vi "TX_双音扫频IMD3.vi"() -> ()   [LabVIEW 2015]
uses:
  <vilib>/Instr/_visa.llb/VISA Configure Serial Port (Instr).vi
  <instrlib>/Agilent E363X Series/Agilent E363X Series.lvlib
  <instrlib>/Rohde&Schwarz Spectrum Analyzer/Rohde&Schwarz Spectrum Analyzer.lvlib
panel:
  out "VISA resource name out 2":refnum<visa-resource-name>
  out "VISA resource name out":refnum<visa-resource-name>
  in  "Stop Frequency (0.0) 2":dbl=2130000000.0 caption="Stop Frequency (0.0)" format="%#.9p"
  in  "Start Frequency (0.0) 2":dbl=2000000000.0 caption="Start Frequency (0.0)" format="%#.9p"
  in  "Stop Frequency (0.0)":dbl=2130000000.0 format="%#.9p"
  in  "Start Frequency (0.0)":dbl=2000000000.0 format="%#.9p"
  in  "模板路径 2":path=path "E:/Everst_TestReport/Everst_TestReport_Template.xlsx"
  in  "测试板编号 2":i32=4
  in  "保存路径 2":path=path "E:/Everst_TestReport/Report/Everrst_#"
  in  "开关":bool[](array[boolean])=[FALSE, TRUE, FALSE, TRUE, FALSE, FALSE, FALSE, TRUE, TRUE, FALSE]
  in  "volt2v":dbl[](array[numeric])
  in  "volt1v3":dbl[](array[numeric])
  in  "error in (no error) 6":errorcluster {"code" format="%.0x"}
  in  "error in (no error) 5":errorcluster caption="error in (no error)"
  in  "error in (no error) 4":errorcluster caption="error in (no error)"
  in  "error in (no error) 3":errorcluster
  in  "error in (no error) 2":errorcluster
  in  "error in (no error)":errorcluster
  in  "直流电源2v":refnum<visa-resource-name>="GPIB0::6::INSTR"
  in  "Frequency (1.0e9 Hz)":dbl=10000000.0 format="%.3f"
  in  "RF Output Level (-30.0 dBm)":dbl=10.0 caption="RF Output Level (-30.0)" format="%.3f"
  in  "Reference Level Offset (0.0) 2":dbl=0.95 caption="Reference Level Offset (0.0)" format="%^.3e"
  in  "Coupling Value (0.0) 2":dbl=2000.0 caption="Coupling Value (0.0)" format="%^.3e"
  in  "Reference Level (-20.0) 2":dbl=30.0 caption="Reference Level (-20.0)" format="%^.3e"
  in  "Span (0.0) 2":dbl=1000000000.0 caption="Span (0.0)" format="%.1f"
  in  "Center Frequency (0.0) 2":dbl=2100000000.0 caption="Center Frequency (0.0)" format="%#.9p"
  in  "Reference Level Offset (0.0)":dbl=2.3 format="%^.3e"
  in  "Coupling Value (0.0)":dbl=2000.0 format="%^.3e"
  in  "Reference Level (-20.0)":dbl=30.0 format="%^.3e"
  in  "Span (0.0)":dbl=1000000000.0 format="%.1f"
  in  "Center Frequency (0.0)":dbl=2100000000.0 format="%#.9p"
  in  "配置文件路径":path=path "E:/Everst_TestReport/config.xlsx"
  out "Bamp_next":dbl[](array[numeric])
  out "Bamp_max":dbl[](array[numeric])
  in  "Marker Search 4":i32(ring)=1 caption="Marker Search" items=["Peak Maximum"=1, "Peak Minimum"=2, "Next Maximum"=3, "Left Maximum"=4, "Right Maximum"=5, "Next Minimum"=6, "Left Minimum"=7, "Right Minimum"=8]
  in  "Peak Excursion 4":dbl=3.0 caption="Peak Excursion" format="%.1f"
  out "channelB_y1":dbl[](array[numeric]) caption="Amplitude" format="%^.3e"
  out "channelB_x1":dbl[](array[numeric]) caption="X" format="%^.3e"
  out "Apos_next":dbl[](array[numeric])
  in  "Aamp_next":dbl[](array[numeric])
  out "Aamp_max":dbl[](array[numeric])
  out "Apos_max":dbl[](array[numeric])
  in  "Marker Search 3":i32(ring)=1 caption="Marker Search" items=["Peak Maximum"=1, "Peak Minimum"=2, "Next Maximum"=3, "Left Maximum"=4, "Right Maximum"=5, "Next Minimum"=6, "Left Minimum"=7, "Right Minimum"=8]
  in  "Peak Excursion 3":dbl=3.0 caption="Peak Excursion" format="%.1f"
  out "channelA_y1":dbl[](array[numeric]) caption="Amplitude" format="%^.3e"
  out "channelA_x1":dbl[](array[numeric]) caption="X" format="%^.3e"
  in  "信号发生器地址":refnum<visa-resource-name>="GPIB0::10::INSTR"
  in  "频谱仪地址B":refnum<visa-resource-name>="TCPIP0::192.168.1.4::inst0::INSTR"
  in  "频谱仪地址A":refnum<visa-resource-name>="GPIB0::22::INSTR"
  in  "直流电源(1.3V)":refnum<visa-resource-name>="GPIB0::4::INSTR"
  in  "FPGA串口地址":refnum<visa-resource-name>="COM3"
  out "fin":dbl[](array[numeric])
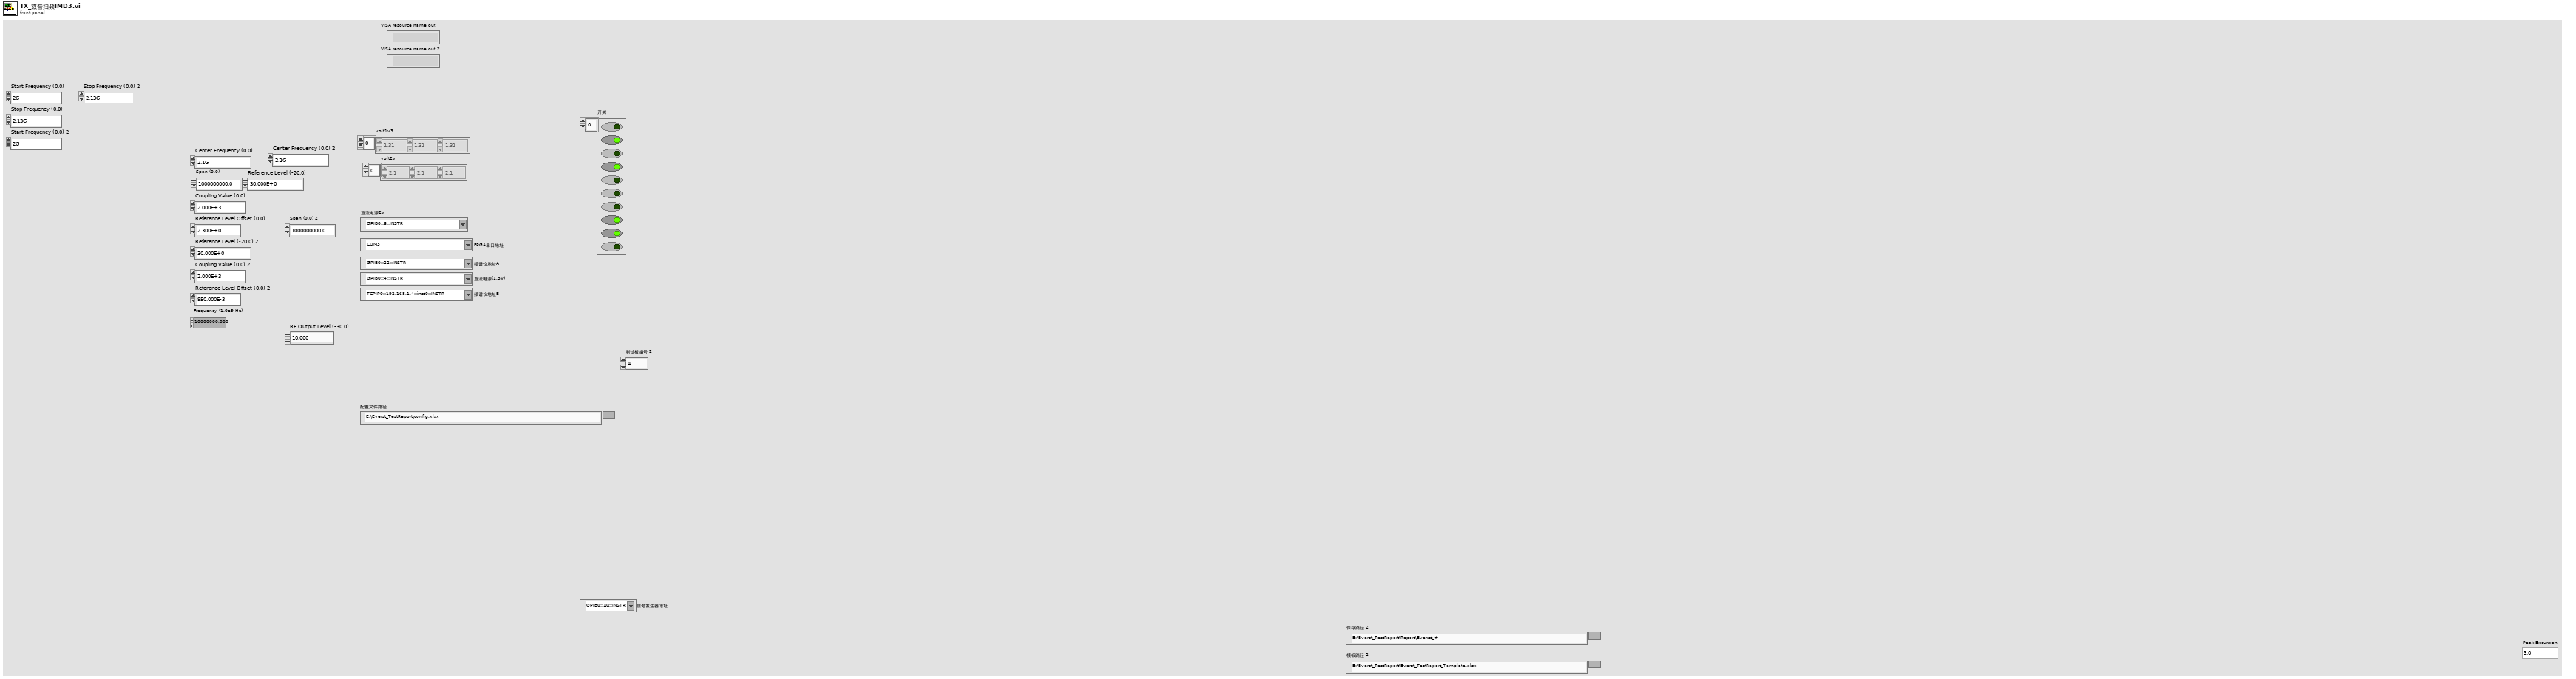
[diagram p1: front panel]
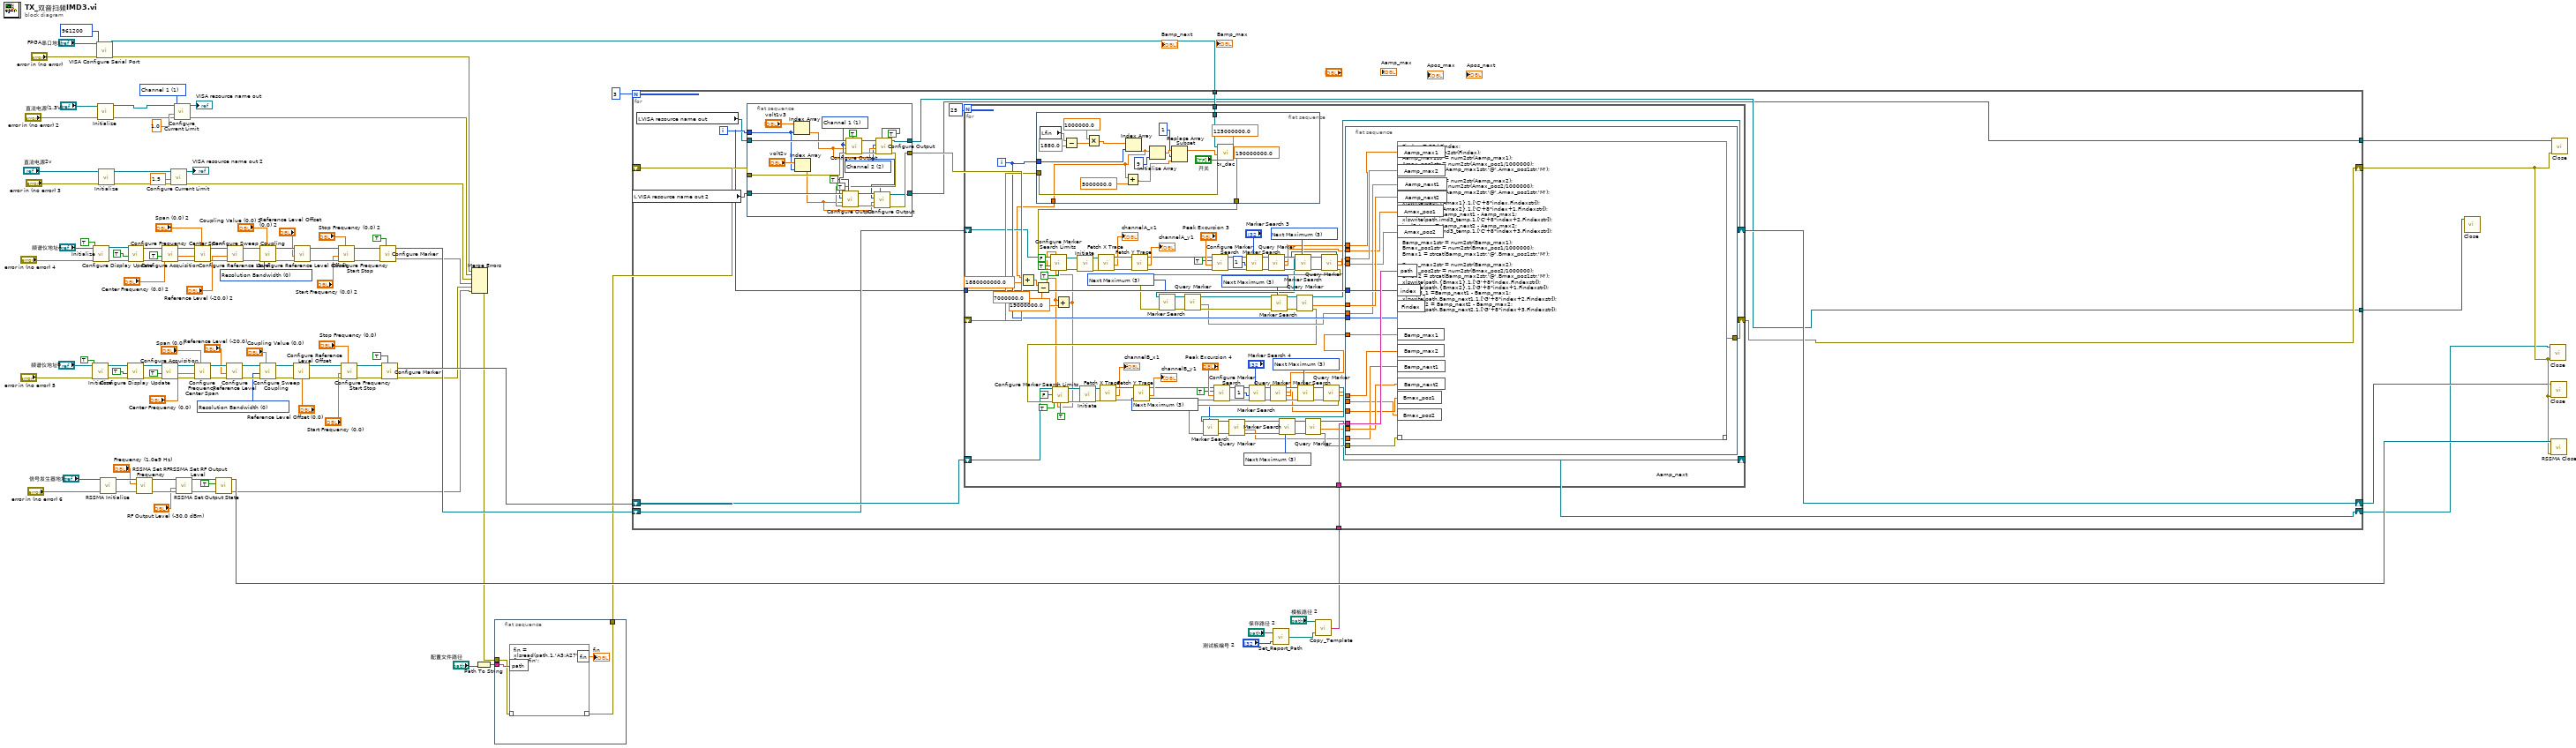
[diagram p0: block diagram]
diagram:
  w42 = 1 items=["Channel 1"=1, "Channel 2"=2, "Channel 3"=3] ("Channel (1: Channel 1)")
  w50 = 0 items=["Resolution Bandwidth", "Video Bandwidth", "Sweep Time"] ("Sweep Coupling (Resolution Bandwidth)")
  w72 = 0 items=["Resolution Bandwidth", "Video Bandwidth", "Sweep Time"] ("Sweep Coupling (Resolution Bandwidth)")
  n1 = call <instrlib>:"Initialize.vi"("VISA resource name"="频谱仪地址B", "Reset (T: Reset)"=TRUE, "error in (no error)"="error in (no error) 5") -> ("VISA resource name out"=w88:refnum<visa-resource-name>, "error out"=w89:errorcluster)  [unwired: 11 in]
  n2 = call <instrlib>:"Initialize.vi"("VISA resource name"="频谱仪地址A", "Reset (T: Reset)"=TRUE, "error in (no error)"="error in (no error) 4") -> ("VISA resource name out"=w66:refnum<visa-resource-name>, "error out"=w67:errorcluster)  [unwired: 11 in]
  n3 = call-poly "VISA Configure Serial Port"("VISA resource name"="FPGA串口地址", "baud rate (9600)"=u32 961200, "error in (no error)"="error in (no error)") -> ("VISA resource name out"=w111:refnum<visa-resource-name>, "error out"=w36:errorcluster)  [unwired: 11 in]
  n4 = call <instrlib>:"Initialize.vi"("error in (no error)"="error in (no error) 2", "VISA resource name"="直流电源(1.3V)") -> ("error out"=w39:errorcluster, "VISA resource name out"=w40:refnum<visa-resource-name>)  [unwired: 8 in]
  n5 = call <instrlib>:"Initialize.vi"("error in (no error)"="error in (no error) 3", "VISA resource name"="直流电源2v") -> ("error out"=w47:errorcluster, "VISA resource name out"=w46:refnum<visa-resource-name>)  [unwired: 8 in]
  n6 = call <instrlib>:"RSSMA Initialize.vi"("error in (no error)"="error in (no error) 6", "Resource Name (GPIB::28)"="信号发生器地址") -> ("error out"=w100:errorcluster, "dup VISA session"=w99:refnum<visa-resource-name>)  [unwired: 8 in]
  n7 = call <instrlib>:"Configure Display Update.vi"("error in (no error)"=w89, "Display In Remote (F: Off)"=TRUE, "VISA resource name"=w88) -> ("error out"=w87:errorcluster, "VISA resource name out"=w86:refnum<visa-resource-name>)  [unwired: 7 in]
  n8 = call <instrlib>:"Configure Display Update.vi"("error in (no error)"=w67, "Display In Remote (F: Off)"=TRUE, "VISA resource name"=w66) -> ("error out"=w65:errorcluster, "VISA resource name out"=w64:refnum<visa-resource-name>)  [unwired: 7 in]
  n9 = call <instrlib>:"RSSMA Set RF Frequency.vi"("error in (no error)"=w100, "Frequency (1.0e9 Hz)"="Frequency (1.0e9 Hz)", "VISA session"=w99) -> ("error out"=w97:errorcluster, "dup VISA session"=w96:refnum<visa-resource-name>)  [unwired: 7 in]
  n10 = call <instrlib>:"Configure Acquisition.vi"("error in (no error)"=w87, "Sweep Mode Continuous (F: Off)"=TRUE, "VISA resource name"=w86) -> ("error out"=w84:errorcluster, "VISA resource name out"=w83:refnum<visa-resource-name>)  [unwired: 7 in]
  n11 = call <instrlib>:"Configure Acquisition.vi"("error in (no error)"=w65, "Sweep Mode Continuous (F: Off)"=TRUE, "VISA resource name"=w64) -> ("error out"=w62:errorcluster, "VISA resource name out"=w61:refnum<visa-resource-name>)  [unwired: 7 in]
  n12 = call <instrlib>:"Configure Current Limit.vi"("error in (no error)"=w47, "Current Limit (0.0 A)"=1.5, "VISA resource name"=w46) -> ("error out"=w34:errorcluster, "VISA resource name out"=→"VISA resource name out 2":refnum<visa-resource-name>)  [unwired: 7 in]
  n13 = call <instrlib>:"Configure Current Limit.vi"("error in (no error)"=w39, "Current Limit (0.0 A)"=1.0, "Channel (1: Channel 1)"=w42, "VISA resource name"=w40) -> ("error out"=w35:errorcluster, "VISA resource name out"=→"VISA resource name out":refnum<visa-resource-name>)  [unwired: 6 in]
  n14 = call <instrlib>:"RSSMA Set RF Output Level.vi"("error in (no error)"=w97, "RF Output Level (-30.0 dBm)"="RF Output Level (-30.0 dBm)", "VISA session"=w96) -> ("error out"=w95:errorcluster, "dup VISA session"=w94:refnum<visa-resource-name>)  [unwired: 7 in]
  n15 = call <instrlib>:"Configure Frequency Center Span.vi"("Span (0.0)"="Span (0.0)", "error in (no error)"=w84, "Center Frequency (0.0)"="Center Frequency (0.0)", "VISA resource name"=w83) -> ("error out"=w82:errorcluster, "VISA resource name out"=w81:refnum<visa-resource-name>)  [unwired: 6 in]
  n16 = call <instrlib>:"Configure Frequency Center Span.vi"("Span (0.0)"="Span (0.0) 2", "error in (no error)"=w62, "Center Frequency (0.0)"="Center Frequency (0.0) 2", "VISA resource name"=w61) -> ("error out"=w60:errorcluster, "VISA resource name out"=w59:refnum<visa-resource-name>)  [unwired: 6 in]
  n17 = call <instrlib>:"RSSMA Set Output State.vi"("error in (no error)"=w95, "RF Output State (F: Off)"=TRUE, "VISA session"=w94) -> ("error out"=w31:errorcluster, "dup VISA session"=w110:refnum<visa-resource-name>)  [unwired: 7 in]
  n18 = call <instrlib>:"Configure Reference Level.vi"("error in (no error)"=w82, "Reference Level (-20.0)"="Reference Level (-20.0)", "VISA resource name"=w81) -> ("error out"=w80:errorcluster, "VISA resource name out"=w79:refnum<visa-resource-name>)  [unwired: 7 in]
  n19 = call <instrlib>:"Configure Reference Level.vi"("error in (no error)"=w60, "Reference Level (-20.0)"="Reference Level (-20.0) 2", "VISA resource name"=w59) -> ("error out"=w58:errorcluster, "VISA resource name out"=w57:refnum<visa-resource-name>)  [unwired: 7 in]
  n20 = call <instrlib>:"Configure Sweep Coupling.vi"("Coupling Value (0.0)"="Coupling Value (0.0)", "error in (no error)"=w80, "Sweep Coupling (Resolution Bandwidth)"=w72, "VISA resource name"=w79) -> ("error out"=w78:errorcluster, "VISA resource name out"=w77:refnum<visa-resource-name>)  [unwired: 6 in]
  n21 = call <instrlib>:"Configure Sweep Coupling.vi"("Coupling Value (0.0)"="Coupling Value (0.0) 2", "error in (no error)"=w58, "Sweep Coupling (Resolution Bandwidth)"=w50, "VISA resource name"=w57) -> ("error out"=w56:errorcluster, "VISA resource name out"=w55:refnum<visa-resource-name>)  [unwired: 6 in]
  n22 = call <instrlib>:"Configure Reference Level Offset.vi"("error in (no error)"=w78, "Reference Level Offset (0.0)"="Reference Level Offset (0.0)", "VISA resource name"=w77) -> ("error out"=w14:errorcluster, "VISA resource name out"=w13:refnum<visa-resource-name>)  [unwired: 7 in]
  n23 = call <instrlib>:"Configure Reference Level Offset.vi"("error in (no error)"=w56, "Reference Level Offset (0.0)"="Reference Level Offset (0.0) 2", "VISA resource name"=w55) -> ("error out"=w18:errorcluster, "VISA resource name out"=w17:refnum<visa-resource-name>)  [unwired: 7 in]
  n24 = call <instrlib>:"Configure Frequency Start Stop.vi"("Stop Frequency (0.0)"="Stop Frequency (0.0) 2", "error in (no error)"=w18, "Start Frequency (0.0)"="Start Frequency (0.0) 2", "VISA resource name"=w17) -> ("error out"=w16:errorcluster, "VISA resource name out"=w15:refnum<visa-resource-name>)  [unwired: 6 in]
  n25 = call <instrlib>:"Configure Frequency Start Stop.vi"("Stop Frequency (0.0)"="Stop Frequency (0.0)", "error in (no error)"=w14, "Start Frequency (0.0)"="Start Frequency (0.0)", "VISA resource name"=w13) -> ("error out"=w12:errorcluster, "VISA resource name out"=w11:refnum<visa-resource-name>)  [unwired: 6 in]
  n26 = call <instrlib>:"Configure Marker.vi"("Marker State (F: Off)"=TRUE, "error in (no error)"=w16, "VISA resource name"=w15) -> ("error out"=w33:errorcluster, "VISA resource name out"=w106:refnum<visa-resource-name>)  [unwired: 7 in]
  n27 = call <instrlib>:"Configure Marker.vi"("Marker State (F: Off)"=TRUE, "error in (no error)"=w12, "VISA resource name"=w11) -> ("error out"=w32:errorcluster, "VISA resource name out"=w107:refnum<visa-resource-name>)  [unwired: 7 in]
  n28 = Merge Errors(w36, w35, w34, w33, w32, w31) -> (w24:errorcluster)
  n29 = Path To String(path="配置文件路径") -> (string=w103:string)
  n30 = flat-sequence {
    tunnel: w103 -> [w115]
    tunnel: w24 -> [w114]
    tunnel: [w113] -> w23
    frame #0 {
      n31 = script code="fin = xlsread(path,1,'A3:A27');\nfin = fin';"("??"=w114, "path"=w115) -> ("??"=w113:errorcluster, "fin"=→"fin":dbl[])
    }
  }
  n32 = call "Set_Report_Path.vi"("测试板编号"="测试板编号 2", "保存路径"="保存路径 2") -> ("创建生成路径"=w21:path)
  n33 = call "Copy_Template.vi"("报告保存路径"=w21, "模板路径"="模板路径 2") -> ("报告保存路径字符串"=w19:string)
  n34 = for {
    N: 3 -> [_]
    tunnel: w111 -> [w131]
    shift-right: [w123] -> w109
    shift-left: w23 -> [w130]
    shift-right: [w129] -> w108
    shift-left: w107 -> [w128]
    shift-right: [w126] -> w105
    shift-left: w106 -> [w127]
    tunnel: w19 -> [w122]
    tunnel: [w118] -> w4
    tunnel: [w117] -> w3
    i -> [w121]
    n35 = local read "VISA resource name out 2"() -> (w119:refnum<visa-resource-name>)
    n36 = local read "VISA resource name out"() -> (w120:refnum<visa-resource-name>)
    n37 = flat-sequence {
      tunnel: w120 -> [w293]
      tunnel: w130 -> [w291]
      tunnel: w119 -> [w290]
      tunnel: [w280] -> w124
      tunnel: [w284] -> w118
      tunnel: [w276] -> w117
      tunnel: w121 -> [w274]
      frame #0 {
        w275 = 2 items=["Channel 1"=1, "Channel 2"=2, "Channel 3"=3] ("Channel (1: Channel 1)")
        w289 = 1 items=["Channel 1"=1, "Channel 2"=2, "Channel 3"=3] ("Channel (1: Channel 1)")
        n38 = Index Array(array="volt1v3", index=w274) -> (element=w279:dbl)
        n39 = Index Array(array="volt2v", index=w274) -> (element=w278:dbl)
        n40 = call <instrlib>:"Configure Output.vi"("Enable Output (T: Enable)"=TRUE, "error in (no error)"=w291, "Voltage Level (0.0 V)"=w279, "Channel (1: Channel 1)"=w289, "VISA resource name"=w293) -> ("error out"=w283:errorcluster, "VISA resource name out"=w285:refnum<visa-resource-name>)  [unwired: 5 in]
        n41 = call <instrlib>:"Configure Output.vi"("Enable Output (T: Enable)"=TRUE, "error in (no error)"=w283, "Voltage Level (0.0 V)"=w279, "Channel (1: Channel 1)"=w275, "VISA resource name"=w285) -> ("error out"=w282:errorcluster, "VISA resource name out"=w284:refnum<visa-resource-name>)  [unwired: 5 in]
        n42 = call <instrlib>:"Configure Output.vi"("Enable Output (T: Enable)"=TRUE, "error in (no error)"=w282, "Voltage Level (0.0 V)"=w278, "Channel (1: Channel 1)"=w289, "VISA resource name"=w290) -> ("error out"=w281:errorcluster, "VISA resource name out"=w277:refnum<visa-resource-name>)  [unwired: 5 in]
        n43 = call <instrlib>:"Configure Output.vi"("Enable Output (T: Enable)"=TRUE, "error in (no error)"=w281, "Voltage Level (0.0 V)"=w278, "Channel (1: Channel 1)"=w275, "VISA resource name"=w277) -> ("error out"=w280:errorcluster, "VISA resource name out"=w276:refnum<visa-resource-name>)  [unwired: 5 in]
      }
    }
    n44 = for {
      N: 25 -> [_]
      tunnel: w131 -> [w235]
      shift-right: [w191] -> w123
      shift-left: w124 -> [w234]
      shift-right: [w185] -> w129
      shift-left: w127 -> [w150]
      shift-right: [w180] -> w126
      shift-left: w128 -> [w138]
      tunnel: w122 -> [w190]
      tunnel: w121 -> [w188]
      i -> [w189]
      w132 = 3 items=["Peak Maximum"=1, "Peak Minimum"=2, "Next Maximum"=3, "Left Maximum"=4, "Right Maximum"=5, "Next Minimum"=6, "Left Minimum"=7, "Right Minimum"=8] ("Marker Search (Peak Maximum)")
      w172 = 3 items=["Peak Maximum"=1, "Peak Minimum"=2, "Next Maximum"=3, "Left Maximum"=4, "Right Maximum"=5, "Next Minimum"=6, "Left Minimum"=7, "Right Minimum"=8] ("Marker Search (Peak Maximum)")
      w179 = 3 items=["Peak Maximum"=1, "Peak Minimum"=2, "Next Maximum"=3, "Left Maximum"=4, "Right Maximum"=5, "Next Minimum"=6, "Left Minimum"=7, "Right Minimum"=8] ("Marker Search (Peak Maximum)")
      w184 = 3 items=["Peak Maximum"=1, "Peak Minimum"=2, "Next Maximum"=3, "Left Maximum"=4, "Right Maximum"=5, "Next Minimum"=6, "Left Minimum"=7, "Right Minimum"=8] ("Marker Search (Peak Maximum)")
      w192 = 3 items=["Peak Maximum"=1, "Peak Minimum"=2, "Next Maximum"=3, "Left Maximum"=4, "Right Maximum"=5, "Next Minimum"=6, "Left Minimum"=7, "Right Minimum"=8] ("Marker Search (Peak Maximum)")
      w213 = 3 items=["Peak Maximum"=1, "Peak Minimum"=2, "Next Maximum"=3, "Left Maximum"=4, "Right Maximum"=5, "Next Minimum"=6, "Left Minimum"=7, "Right Minimum"=8] ("Marker Search (Peak Maximum)")
      n45 = Add(x=w148, y=1880000000.0) -> (x+y=w147:dbl)
      n46 = Subtract(x=w147, y=7000000.0) -> (x-y=w133:dbl)
      n47 = flat-sequence {
        tunnel: w189 -> [w269]
        tunnel: w235 -> [w268]
        tunnel: w234 -> [w265]
        tunnel: [w264] -> w153
        tunnel: [w253] -> w148
        frame #0 {
          n48 = local read "fin"() -> (w271:dbl[])
          n49 = Subtract(x=w271, y=1880.0) -> (x-y=w262:dbl[])
          n50 = Multiply(x=1000000.0, y=w262) -> (x*y=w261:dbl[])
          n51 = Index Array(array=w261, index=w269) -> (element=w253:dbl)
          n52 = Add(x=w253, y=5000000.0) -> (x+y=w254:dbl)
          n53 = Initialize Array(w253, 9 ("dimension size")) -> (w258:dbl[])
          n54 = Replace Array Subset(array=w258, new element=w254, index=1) -> (w257:dbl[])
          n55 = call "tx_dac.vi"("fnco"=190000000.0, "fs"=125000000.0, "error in (no error)"=w265, "fin"=w257, "开关"="开关", "VISA resource name 2"=w268) -> ("error out"=w264:errorcluster)
        }
      }
      n56 = Add(x=w133, y=19000000.0) -> (x+y=w134:dbl)
      n57 = call <instrlib>:"Configure Marker Search Limits.vi"("VISA resource name"=w150, "Search Limit Left (0.0)"=w133, "Threshold State (T: On)"=FALSE, "Search Limits (F: Off)"=TRUE, "error in (no error)"=w153, "Search Limit Right (0.0)"=w134, "Search Limits Zoom (F: Off)"=TRUE) -> ("VISA resource name out"=w151:refnum<visa-resource-name>, "error out"=w152:errorcluster)  [unwired: 7 in]
      n58 = call <instrlib>:"Initiate.vi"("error in (no error)"=w152, "VISA resource name"=w151) -> ("error out"=w218:errorcluster, "VISA resource name out"=w219:refnum<visa-resource-name>)  [unwired: 8 in]
      n59 = call <instrlib>:"Fetch X Trace.vi"("error in (no error)"=w218, "VISA resource name"=w219) -> ("error out"=w232:errorcluster, "X"=→"channelA_x1":dbl[], "VISA resource name out"=w233:refnum<visa-resource-name>)  [unwired: 7 in]
      n60 = call <instrlib>:"Fetch Y Trace.vi"("error in (no error)"=w232, "VISA resource name"=w233) -> ("error out"=w220:errorcluster, "Amplitude"=→"channelA_y1":dbl[], "VISA resource name out"=w221:refnum<visa-resource-name>)  [unwired: 7 in]
      n61 = call <instrlib>:"Configure Marker Search.vi"("error in (no error)"=w220, "Peak Excursion (6.0)"="Peak Excursion 3", "Local Oscillator Supression (T: On)"=TRUE ("Local Oscillator Supression (On)"), "VISA resource name"=w221) -> ("error out"=w226:errorcluster, "VISA resource name out"=w225:refnum<visa-resource-name>)  [unwired: 6 in]
      n62 = call <instrlib>:"Marker Search.vi"("Marker Search (Peak Maximum)"="Marker Search 3", "error in (no error)"=w226, "Marker (1)"=1, "VISA resource name"=w225) -> ("error out"=w223:errorcluster, "VISA resource name out"=w224:refnum<visa-resource-name>)  [unwired: 6 in]
      n63 = call <instrlib>:"Query Marker.vi"("error in (no error)"=w223, "VISA resource name"=w224) -> ("error out"=w217:errorcluster, "Marker Amplitude"=w168:dbl, "Marker Position"=w167:dbl, "VISA resource name out"=w216:refnum<visa-resource-name>)  [unwired: 6 in]
      n64 = call <instrlib>:"Marker Search.vi"("Marker Search (Peak Maximum)"=w213, "error in (no error)"=w217, "VISA resource name"=w216) -> ("error out"=w215:errorcluster, "VISA resource name out"=w214:refnum<visa-resource-name>)  [unwired: 7 in]
      n65 = call <instrlib>:"Query Marker.vi"("error in (no error)"=w215, "VISA resource name"=w214) -> ("error out"=w178:errorcluster, "Marker Amplitude"=w169:dbl, "Marker Position"=w166:dbl, "VISA resource name out"=w175:refnum<visa-resource-name>)  [unwired: 6 in]
      n66 = call <instrlib>:"Marker Search.vi"("Marker Search (Peak Maximum)"=w172, "error in (no error)"=w178, "VISA resource name"=w175) -> ("error out"=w177:errorcluster, "VISA resource name out"=w174:refnum<visa-resource-name>)  [unwired: 7 in]
      n67 = call <instrlib>:"Query Marker.vi"("error in (no error)"=w177, "VISA resource name"=w174) -> ("error out"=w176:errorcluster, "Marker Amplitude"=w170:dbl, "VISA resource name out"=w173:refnum<visa-resource-name>)  [unwired: 6 in, 1 out]
      n68 = call <instrlib>:"Marker Search.vi"("Marker Search (Peak Maximum)"=w184, "error in (no error)"=w176, "VISA resource name"=w173) -> ("error out"=w187:errorcluster, "VISA resource name out"=w186:refnum<visa-resource-name>)  [unwired: 7 in]
      n69 = call <instrlib>:"Query Marker.vi"("error in (no error)"=w187, "VISA resource name"=w186) -> ("error out"=w141:errorcluster, "Marker Amplitude"=w171:dbl, "VISA resource name out"=w185:refnum<visa-resource-name>)  [unwired: 6 in, 1 out]
      n70 = call <instrlib>:"Configure Marker Search Limits.vi"("VISA resource name"=w138, "Search Limit Left (0.0)"=w133, "Threshold State (T: On)"=FALSE, "Search Limits (F: Off)"=TRUE, "error in (no error)"=w141, "Search Limit Right (0.0)"=w134, "Search Limits Zoom (F: Off)"=TRUE) -> ("VISA resource name out"=w140:refnum<visa-resource-name>, "error out"=w139:errorcluster)  [unwired: 7 in]
      n71 = call <instrlib>:"Initiate.vi"("error in (no error)"=w139, "VISA resource name"=w140) -> ("error out"=w197:errorcluster, "VISA resource name out"=w198:refnum<visa-resource-name>)  [unwired: 8 in]
      n72 = call <instrlib>:"Fetch X Trace.vi"("error in (no error)"=w197, "VISA resource name"=w198) -> ("error out"=w211:errorcluster, "X"=→"channelB_x1":dbl[], "VISA resource name out"=w212:refnum<visa-resource-name>)  [unwired: 7 in]
      n73 = call <instrlib>:"Fetch Y Trace.vi"("error in (no error)"=w211, "VISA resource name"=w212) -> ("error out"=w199:errorcluster, "Amplitude"=→"channelB_y1":dbl[], "VISA resource name out"=w200:refnum<visa-resource-name>)  [unwired: 7 in]
      n74 = call <instrlib>:"Configure Marker Search.vi"("error in (no error)"=w199, "Peak Excursion (6.0)"="Peak Excursion 4", "Local Oscillator Supression (T: On)"=TRUE ("Local Oscillator Supression (On)"), "VISA resource name"=w200) -> ("error out"=w205:errorcluster, "VISA resource name out"=w204:refnum<visa-resource-name>)  [unwired: 6 in]
      n75 = call <instrlib>:"Marker Search.vi"("Marker Search (Peak Maximum)"="Marker Search 4", "error in (no error)"=w205, "Marker (1)"=1, "VISA resource name"=w204) -> ("error out"=w202:errorcluster, "VISA resource name out"=w203:refnum<visa-resource-name>)  [unwired: 6 in]
      n76 = call <instrlib>:"Query Marker.vi"("error in (no error)"=w202, "VISA resource name"=w203) -> ("error out"=w196:errorcluster, "Marker Amplitude"=w165:dbl, "Marker Position"=w155:dbl, "VISA resource name out"=w195:refnum<visa-resource-name>)  [unwired: 6 in]
      n77 = call <instrlib>:"Marker Search.vi"("Marker Search (Peak Maximum)"=w192, "error in (no error)"=w196, "VISA resource name"=w195) -> ("error out"=w194:errorcluster, "VISA resource name out"=w193:refnum<visa-resource-name>)  [unwired: 7 in]
      n78 = call <instrlib>:"Query Marker.vi"("error in (no error)"=w194, "VISA resource name"=w193) -> ("error out"=w163:errorcluster, "Marker Amplitude"=w156:dbl, "Marker Position"=w154:dbl, "VISA resource name out"=w164:refnum<visa-resource-name>)  [unwired: 6 in]
      n79 = call <instrlib>:"Marker Search.vi"("Marker Search (Peak Maximum)"=w132, "error in (no error)"=w163, "VISA resource name"=w164) -> ("error out"=w162:errorcluster, "VISA resource name out"=w160:refnum<visa-resource-name>)  [unwired: 7 in]
      n80 = call <instrlib>:"Query Marker.vi"("error in (no error)"=w162, "VISA resource name"=w160) -> ("error out"=w161:errorcluster, "Marker Amplitude"=w157:dbl, "VISA resource name out"=w159:refnum<visa-resource-name>)  [unwired: 6 in, 1 out]
      n81 = call <instrlib>:"Marker Search.vi"("Marker Search (Peak Maximum)"=w179, "error in (no error)"=w161, "VISA resource name"=w159) -> ("error out"=w183:errorcluster, "VISA resource name out"=w182:refnum<visa-resource-name>)  [unwired: 7 in]
      n82 = call <instrlib>:"Query Marker.vi"("error in (no error)"=w183, "VISA resource name"=w182) -> ("error out"=w181:errorcluster, "Marker Amplitude"=w158:dbl, "VISA resource name out"=w180:refnum<visa-resource-name>)  [unwired: 6 in, 1 out]
      n83 = flat-sequence {
        tunnel: [w252] -> w191
        tunnel: w190 -> [w251]
        tunnel: w189 -> [w250]
        tunnel: w188 -> [w249]
        tunnel: w181 -> [w248]
        tunnel: w171 -> [w247]
        tunnel: w170 -> [w246]
        tunnel: w169 -> [w245]
        tunnel: w168 -> [w244]
        tunnel: w167 -> [w243]
        tunnel: w166 -> [w242]
        tunnel: w165 -> [w241]
        tunnel: w158 -> [w240]
        tunnel: w157 -> [w239]
        tunnel: w156 -> [w238]
        tunnel: w155 -> [w237]
        tunnel: w154 -> [w236]
        frame #0 {
          n84 = script code="Findex = 35+Findex;\nFindexstr = num2str(Findex);\nAamp_max1str = num2str(Aamp_max1);\nAmax_pos1str = num2str(Amax_pos1/1000000);\nAmax1 = strcat(Aamp_max1str,'@',Amax_pos1str,'M');\n\nAamp_max2str = num2str(Aamp_max2);\nAmax_pos2str = num2str(Amax_pos2/1000000);\nAmax2 = strcat(Aamp_max2str,'@',Amax_pos1str,'M');\n\nxlswrite(path,{Amax1},1,['C'+8*index,Findexstr]);\nxlswrite(path,{Amax2},1,['C'+8*index+1,Findexstr]);\nimd3_temp = Aamp_next1 - Aamp_max1;\nxlswrite(path,imd3_temp,1,['C'+8*index+2,Findexstr]);\nimd3_temp = Aamp_next2 - Aamp_max2;\nxlswrite(path,imd3_temp,1,['C'+8*index+3,Findexstr]);\n\nBamp_max1str = num2str(Bamp_max1);\nBmax_pos1str = num2str(Bmax_pos1/1000000);\nBmax1 = strcat(Bamp_max1str,'@',Bmax_pos1str,'M');\n\nBamp_max2str = num2str(Bamp_max2);\nBmax_pos2str = num2str(Bmax_pos2/1000000);\nBmax2 = strcat(Bamp_max2str,'@',Bmax_pos1str,'M');\nxlswrite(path,{Bmax1},1,['G'+8*index,Findexstr]);\nxlswrite(path,{Bmax2},1,['G'+8*index+1,Findexstr]);\nb_imd3_1 =Bamp_next1 - Bamp_max1;\nxlswrite(path,Bamp_next1,1,['G'+8*index+2,Findexstr]);\nb_imd3_2 = Bamp_next2 - Bamp_max2;\nxlswrite(path,Bamp_next2,1,['G'+8*index+3,Findexstr]);"("??"=w248, "Aamp_max2"=w245, "path"=w251, "index"=w249, "Bamp_next1"=w239, "Findex"=w250, "Aamp_max1"=w244, "Aamp_next1"=w246, "Aamp_next2"=w247, "Bamp_max1"=w241, "Bamp_max2"=w238, "Bamp_next2"=w240, "Amax_pos1"=w243, "Amax_pos2"=w242, "Bmax_pos1"=w237, "Bmax_pos2"=w236) -> ("??"=w252:errorcluster)
        }
      }
    }
  }
  n85 = call <instrlib>:"Close.vi"("VISA resource name"=w4) -> ()  [unwired: 10 in, 1 out]
  n86 = call <instrlib>:"Close.vi"("error in (no error)"=w109, "VISA resource name"=w105) -> ()  [unwired: 9 in, 1 out]
  n87 = call <instrlib>:"Close.vi"("error in (no error)"=w109, "VISA resource name"=w108) -> ()  [unwired: 9 in, 1 out]
  n88 = call <instrlib>:"RSSMA Close.vi"("error in (no error)"=w109, "VISA session"=w110) -> ()  [unwired: 9 in, 1 out]
  n89 = call <instrlib>:"Close.vi"("error in (no error)"=w109, "VISA resource name"=w3) -> ()  [unwired: 9 in, 1 out]
